vi "Mouse RightDown.vi"(8 "error in (no error)":errorcluster, 9 "Cell Position":T2, 10 "Coords":T1, 11 "MCLB_Template in":refnum<class "MCLB_Template.lvclass">) -> (0 "error out":errorcluster, 3 "MCLB_Template out":refnum<class "MCLB_Template.lvclass">)   [LabVIEW 2021, in "MCLB_Template.lvclass"]
uses:
  MCLB_Template.lvclass
  <vilib>/Utility/miscctls.llb/LVRowAndColumnTypeDef.ctl
  <vilib>/Utility/miscctls.llb/LVPoint32TypeDef.ctl
  MCLB_Template.lvclass/MCLB_Template.ctl
panel:
  out "Coords 2":T1
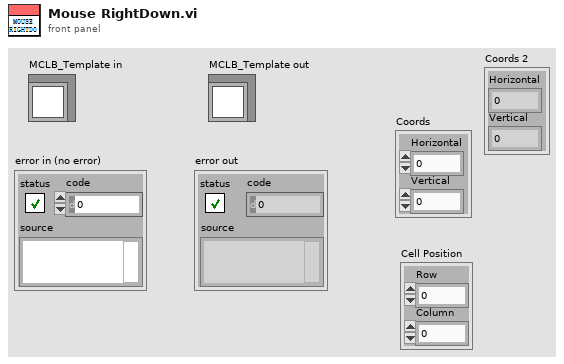
[diagram p1: front panel]
types:
  T1 = typedef "LVPoint32TypeDef.ctl" = cluster{"Horizontal":i32, "Vertical":i32}
  T2 = typedef "LVRowAndColumnTypeDef.ctl" = cluster{"Row":i32, "Column":i32}
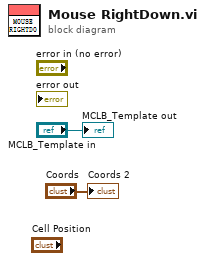
[diagram p0: block diagram]
diagram:
  "MCLB_Template out" <- "MCLB_Template in"
  "Coords 2" <- "Coords"
